vi "Fetch SensorID.vi"(7 "Message":string="Fetch Model Numbers", 8 "error in (no error)":errorcluster, 10 "MSG FetchSensorID Payload in":T1, 11 "Database in":refnum<queue>) -> (0 "error out":errorcluster, 2 "MSG FetchSensorID Payload out":T1, 3 "Database out":refnum<queue>)   [LabVIEW 2026, in "Settings.lvlib"]
uses:
  Architecture/Message Queue/Message Cluster.ctl
  controls/Messaging Payloads/MSG FetchSensorID Payload.ctl
  controls/Messaging Payloads/Fetch SensorID Payload.ctl
  Architecture/Message Queue/Enqueue Message (Single).vi
  Settings/Settings.lvlib
  Architecture/Message Queue/Message Queue.lvlib
  Database/Database.lvlib
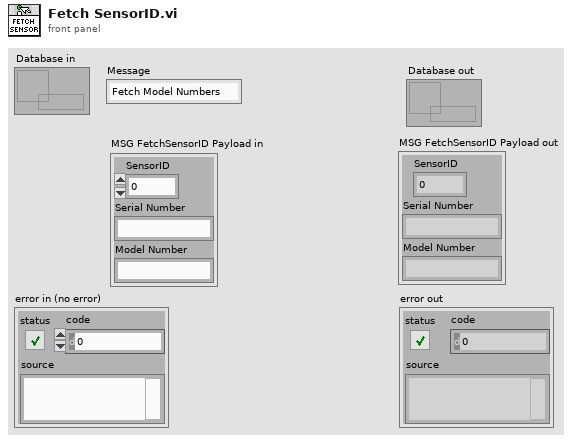
[diagram p1: front panel]
types:
  T1 = typedef "Database.lvlib/MSG FetchSensorID Payload.ctl" = cluster{"SensorID":i32, "Serial Number":string, "Model Number":string}
  T2 = typedef "Database.lvlib/Fetch SensorID Payload.ctl" = cluster{"Notifier":refnum<notifier>, "MSG FetchSensorID Payload":T1}
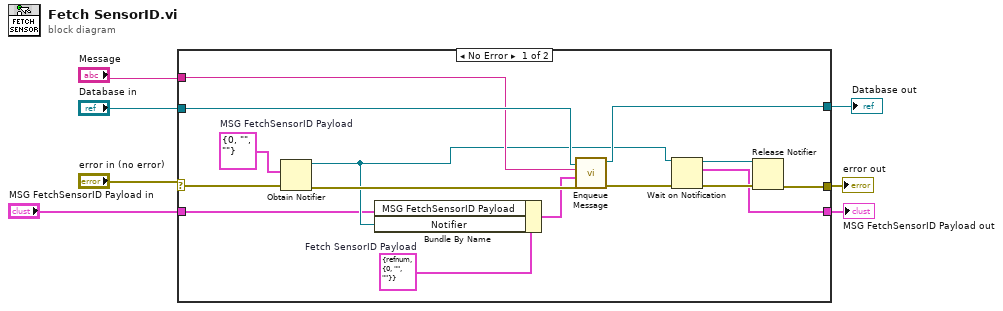
[diagram p0: block diagram]
diagram:
  n1 = case shown="No Error" "error in (no error)" {
    selector: "error in (no error)" -> [w15 w24]
    tunnel: [w22 w25] -> w7
    tunnel: "Database in" -> [w21 w25]
    tunnel: [w20 w24] -> w5
    tunnel: "Message" -> [w12 _]
    tunnel: [w11 w23] -> w1
    tunnel: "MSG FetchSensorID Payload in" -> [w8 w23]
    frame No Error {
      w10 = T1 {"SensorID"=0, "Serial Number"="", "Model Number"=""}  # MSG FetchSensorID Payload
      w14 = T2 {"Notifier"=refnum, "MSG FetchSensorID Payload"={"SensorID"=0, "Serial Number"="", "Model Number"=""}}  # Fetch SensorID Payload
      n2 = Obtain Notifier(notification data type=w10, error in (no error)=w15) -> (notifier out=w9:refnum<notifier>, error out=w16:errorcluster)  [unwired: 2 in, 1 out]
      n3 = Bundle By Name(cluster=w14, "MSG FetchSensorID Payload"=w8, "Notifier"=w9) -> (w13:T2)
      n4 = call-poly "Enqueue Message.vi"("error in (no error)"=w16, "Message Data"=w13, "Message"=w12, "Message Queue"=w21) -> ("error out"=w17:errorcluster, "dup Message Queue"=w22:refnum<queue>)  [unwired: 6 in]
      n5 = Wait on Notification(notifier=w9, error in (no error)=w17) -> (notifier out=w19:refnum<notifier>, notification=w11:T1, error out=w18:errorcluster)  [unwired: 2 in, 1 out]
      n6 = Release Notifier(notifier=w19, error in (no error)=w18) -> (error out=w20:errorcluster)  [unwired: 1 in, 2 out]
    }
    frame Error {
    }
  }
  "Database out" <- w7
  "error out" <- w5
  "MSG FetchSensorID Payload out" <- w1
